vi "Init.vi"(8 "Path":path, 9 "Register":refnum<event-registration>, 10 "Addresses Strategy":refnum<class "Addresses Strategy.lvclass">) -> (3 "jettl Actor out":refnum<class "jettl Actor.lvclass">)   [LabVIEW 2021, in "jettl.lvlib" / "Temporary Actor.lvlib" / "jettl Actor.lvclass"]
uses:
  jettl Actor.lvclass
  Addresses Strategy/Addresses Strategy/Addresses Strategy.lvclass
  Msg/Msg.lvclass
  jettl Actor.lvclass/jettl Actor.ctl
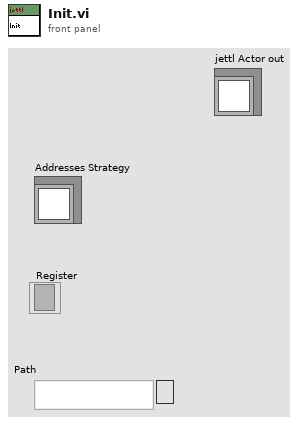
[diagram p1: front panel]
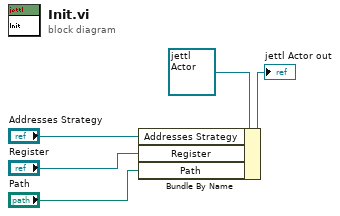
[diagram p0: block diagram]
diagram:
  n1 = Bundle By Name(cluster=refnum<class "jettl Actor.lvclass"> refnum ("jettl Event Actor out"), "Addresses Strategy"="Addresses Strategy", "Register"="Register", "Path"="Path") -> (→"jettl Actor out":refnum<class "jettl Actor.lvclass">)
